vi "SHA-3 Number of Rounds.vi"(1 "Hash Function in":refnum<class "NI_SHA-3.lvclass">) -> (0 "rounds":i32)   [LabVIEW 2020, in "NI_SHA-3.lvclass"]
doc: "Returns the \"Nr\" constant as defined in FIPS PUB 202 for the SHA-3 family of hash functions."
uses:
  <vilib>/security/Message Digest/SHA-3/NI_SHA-3.lvclass
  de10eb19-ecc6-40a5-873c-159babf1c20e.vi
  <vilib>/security/Message Digest/SHA-3/subVIs/Get Word Type.vi
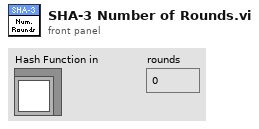
[diagram p1: front panel]
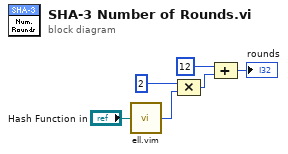
[diagram p0: block diagram]
diagram:
  n1 = call "ell.vim"("Hash Function in"="Hash Function in") -> ("ell"=w3:i32)
  n2 = Compound Arithmetic op=MULTIPLY(2, w3) -> (w5:i32)
  n3 = Compound Arithmetic op=ADD(12, w5) -> (→"rounds":i32)
